vi "Shift Register - Addition of n Numbers.vi"() -> ()   [LabVIEW 2016]
panel:
  in  "Input":i32
  out "Output":i32
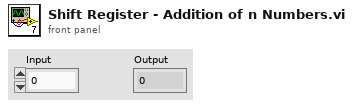
[diagram p1: front panel]
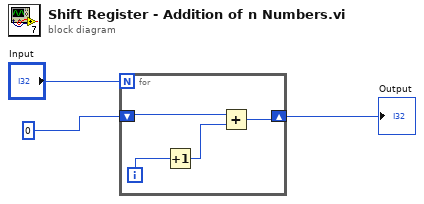
[diagram p0: block diagram]
diagram:
  n1 = for {
    N: "Input" -> [_]
    shift-right: [w5] -> w3
    shift-left: 0 -> [w4]
    i -> [w7]
    n2 = Increment(x=w7) -> (x+1=w6:i32)
    n3 = Add(x=w4, y=w6) -> (x+y=w5:i32)
  }
  "Output" <- w3
